vi "Clear All Discretes.vi"(8 "error in":errorcluster, 11 "FPGA-DIO in":refnum<class "FPGA_DIO.lvclass">) -> (0 "error out":errorcluster, 3 "FPGA-DIO out":refnum<class "FPGA_DIO.lvclass">)   [LabVIEW 2019, in "FPGA_DIO.lvlib" / "FPGA_DIO.lvclass"]
uses:
  Library/FPGA_DIO.lvclass
  C:/Users/Public/Documents/Development/builds/Instruments/DIG_IO.lvlibp/Library/DIG_IO.lvclass
  Library/FPGA_DIO.lvclass/FPGA_DIO.ctl
  builds/Instruments/DIG_IO.lvlibp/Accessors/Read Banks.vi
  builds/Instruments/DIG_IO.lvlibp/Library/DIG_IO.lvclass
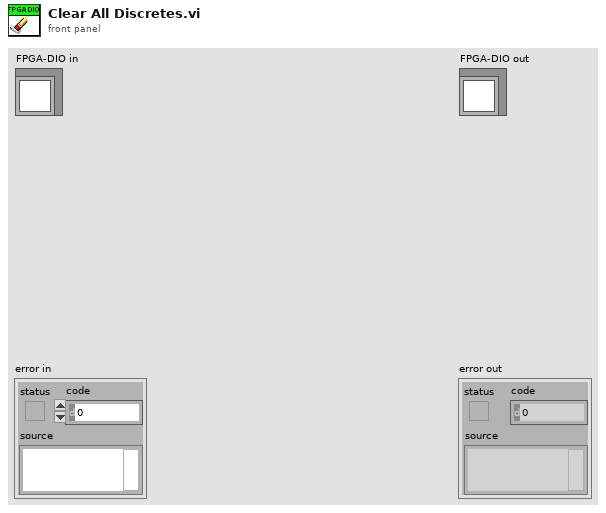
[diagram p1: front panel]
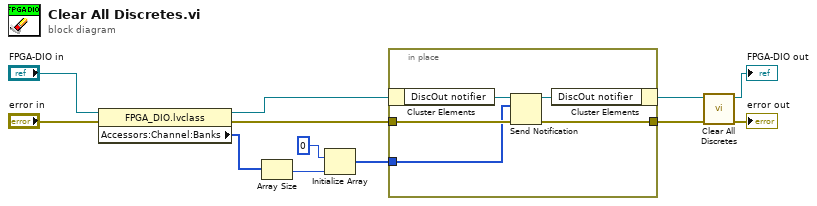
[diagram p0: block diagram]
diagram:
  n1 = property class="FPGA_DIO.lvclass"(reference="FPGA-DIO in", error in="error in") -> (reference out=w5:refnum<class "FPGA_DIO.lvclass">, error out=w3:errorcluster, "Accessors:Channel:Banks"=w8:u8[])
  n2 = Array Size(array=w8) -> (size(s)=w7:i32)
  n3 = Initialize Array(u8 0, w7) -> (w2:u8[])
  n4 = in-place {
    in-place-border: w3 -> [w15]
    in-place-border: w2 -> [w14]
    in-place-border: [w13] -> w1
    n5 = in-place-cluster #1(w5) -> ("DiscOut notifier"=w17:refnum<notifier>)
    n6 = Send Notification(notification=w14, notifier=w17, error in (no error)=w15) -> (notifier out=w16:refnum<notifier>, error out=w13:errorcluster)
    n7 = in-place-cluster #1("DiscOut notifier"=w16) -> (w4:refnum<class "FPGA_DIO.lvclass">)
  }
  n8 = call-parent "Clear All Discretes.vi"("error in"=w1, "DIG_IO in"=w4) -> ("error out"=→"error out":errorcluster, "DIG_IO out"=→"FPGA-DIO out":refnum<class "FPGA_DIO.lvclass">)  [unwired: 8 in]
